vi "Get Forecast Minutely Data.vi"(8 "error in (no error)":errorcluster, 11 "API Output":string) -> (0 "error out":errorcluster, 2 "Minutely Data":T1 {"minutely"."data"."time" format="%#_10g"}, 3 "API Output (copy)":string)   [LabVIEW 2017, in "Dark Sky Weather Data for LabVIEW.lvlib"]
doc: "Parses the Dark Sky API's output for weather data, by the minute, for the next hour"
uses:
  Dark Sky Weather Data for LabVIEW.lvlib
  Controls/Forecast Minutely Data.ctl
  <vilib>/addons/_JKI.lib/Serialization/JSON/JKI JSON Serialization.lvlib
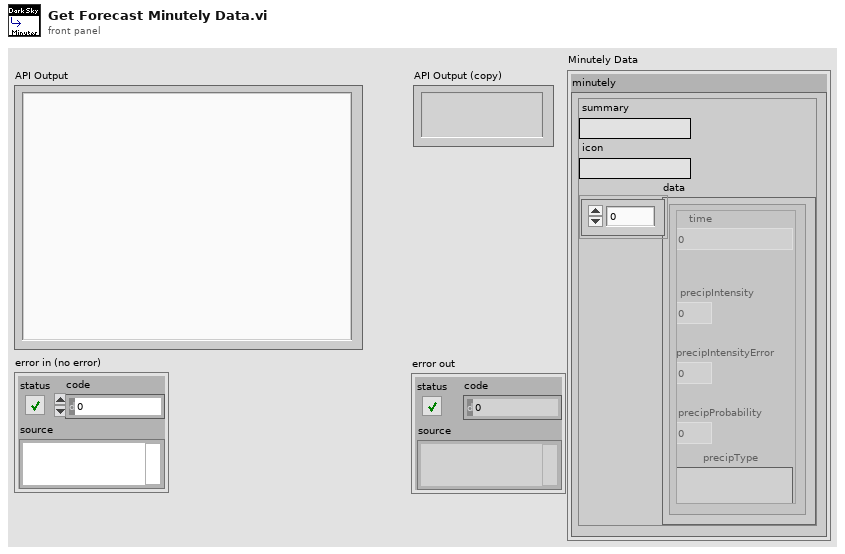
[diagram p1: front panel]
types:
  T1 = typedef "Dark Sky Weather Data for LabVIEW.lvlib/Forecast Minutely Data.ctl" = cluster{"minutely":cluster{"summary":string, "icon":string, "data":cluster{"time":dbl, "precipIntensity":dbl, "precipIntensityError":dbl, "precipProbability":dbl, "precipType":string}[]}}
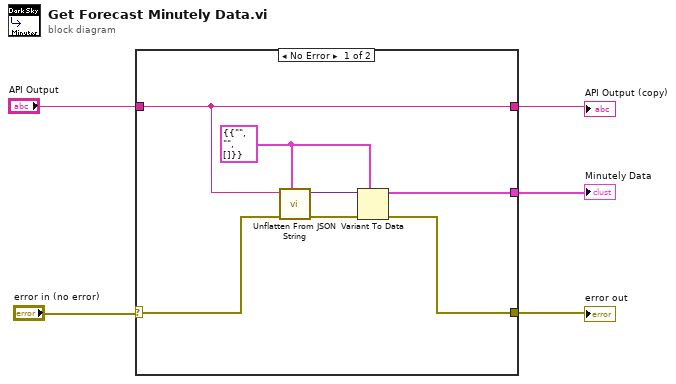
[diagram p0: block diagram]
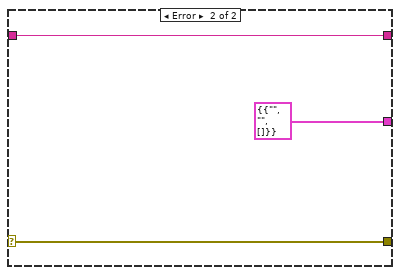
[diagram p2: hidden frame]
diagram:
  n1 = case shown="No Error" "error in (no error)" {
    selector: "error in (no error)" -> [w12 w15]
    tunnel: [w9 w15] -> w4
    tunnel: "API Output" -> [w8 w14]
    tunnel: [w8 w14] -> w2
    tunnel: [w6 T1 {"minutely"={"summary"="", "icon"="", "data"=[]}} ("Minutely Data")] -> w1
    frame No Error {
      w7 = T1 {"minutely"={"summary"="", "icon"="", "data"=[]}} ("Minutely Data")
      n2 = call <vilib>:"Unflatten From JSON String.vi"("Type and Defaults"=w7, "error in (no error)"=w12, "JSON String"=w8) -> ("error out"=w10:errorcluster, "Variant"=w11:variant)  [unwired: 7 in]
      n3 = Variant To Data(error in=w10, type=w7, Variant=w11) -> (data=w6:T1, error out=w9:errorcluster)
    }
    frame Error {
    }
  }
  "error out" <- w4
  "API Output (copy)" <- w2
  "Minutely Data" <- w1
